vi "Write Address.vi"(8 "error in (no error)":errorcluster, 10 "Address":string, 11 "Register Client MSG in":refnum<class "Register Client MSG.lvclass">) -> (0 "error out":errorcluster, 3 "Register Client MSG out":refnum<class "Register Client MSG.lvclass">)   [LabVIEW 2014, in "Register Client MSG.lvclass"]
uses:
  Register Client MSG.lvclass
  Register Client MSG.lvclass/Register Client MSG.ctl
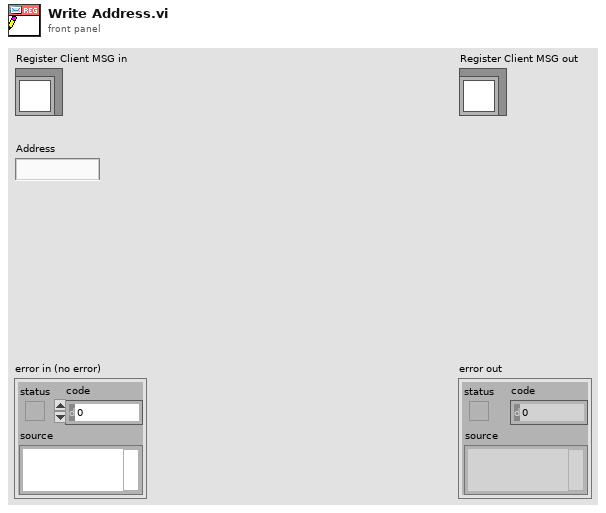
[diagram p1: front panel]
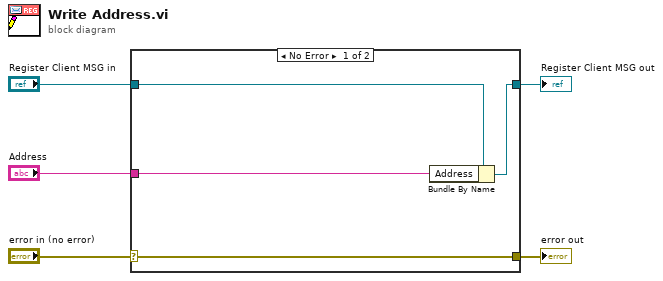
[diagram p0: block diagram]
diagram:
  n1 = case shown="No Error" "error in (no error)" {
    selector: "error in (no error)" -> [w9 w10]
    tunnel: [w9 w10] -> w4
    tunnel: [w7 w11] -> w2
    tunnel: "Register Client MSG in" -> [w8 w11]
    tunnel: "Address" -> [w6 _]
    frame No Error {
      n2 = Bundle By Name(cluster=w8, "Address"=w6) -> (w7:refnum<class "Register Client MSG.lvclass">)
    }
    frame Error {
    }
  }
  "error out" <- w4
  "Register Client MSG out" <- w2
